vi "initMcode.vi"(5 "PinMode":T1, 6 "CheckMenu":bool, 7 "PinControl":T2=4 items=["4"=4, "10"=10, "13"=13, "14"=14, "15"=15, "53"=53, "54"=54, "55"=55, "56"=56, "57"=57, "58"=58, "66"=66, "67"=67, "68"=68, "69"=69, "77"=77, "78"=78], 8 "error in (no error)":errorcluster, 9 "mCode":T3, 10 "DataVariant":variant, 11 "XuLyDataDisplay in":refnum<class "XuLyDataDisplay.lvclass">) -> (0 "error out":errorcluster, 1 "McodeOut":string, 3 "XuLyDataDisplay out":refnum<class "XuLyDataDisplay.lvclass">)   [LabVIEW 2014, in "LibraryGcode.lvlib" / "XuLyDataDisplay.lvclass"]
uses:
  XuLyDataDisplay.lvclass
  SelectMcode.ctl
  PinControl.ctl
  PinMode.ctl
panel:
  in  "StartingAcceleration":cluster{"P":dbl, "R":dbl, "T":dbl}
  in  "MaxAccel":cluster{"X":dbl, "Y":dbl, "Z":dbl}
  in  "StepPerUnit":cluster{"X":dbl, "Y":dbl, "Z":dbl}
  in  "MaxFeedrate":cluster{"X":dbl, "Y":dbl, "Z":dbl}
  in  "PWM_Out":dbl
  in  "StateBoolean":bool
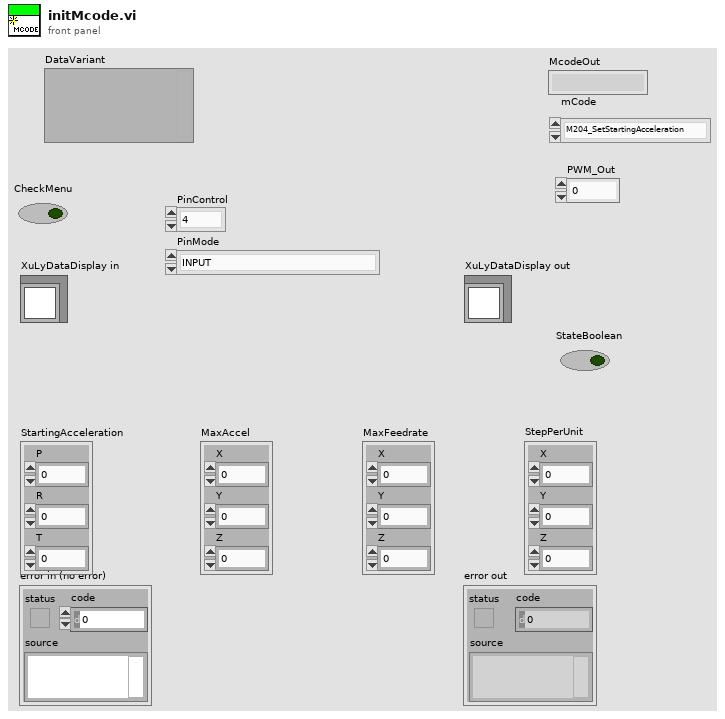
[diagram p1: front panel]
types:
  T1 = typedef "LibraryGcode.lvlib/XuLyDataDisplay.lvclass/PinMode.ctl" = enum16{"INPUT", "OUTPUT", "INPUT_PULLUP", "INPUT_PULLDOWN"}
  T2 = typedef "LibraryGcode.lvlib/XuLyDataDisplay.lvclass/PinControl.ctl" = u16
  T3 = typedef "LibraryGcode.lvlib/XuLyDataDisplay.lvclass/SelectMcode.ctl" = enum16{"M204_SetStartingAcceleration", "M503_ReportSetting", "M500_SaveEprom", "M114_GetPosition", "M92_SetAxisStepPerUnit", "M17_EnableStep", "M18_DisableStep", "M80_PowerOn", "M81_PowerOff", "M112_EMGStop", "M118_SerialPrint", "M226_WaitforPinState", "M400_WaitFinishMove", "M203_SetMaxFeedRate", "M201_SetMaxACCEL", "M380_381_SetSoleNoid_On_Off", "M42_InitPin", "M42_PinControl", "M106_SetFan1", "M106_SetFan2", "M106_SetFan3", "M3_SetSpindle", "M5_OffSpindle", "M999_RestartStop"}
  T4 = typedef "LibraryGcode.lvlib/TypeFirmwareControl.ctl" = enum16{"ScaraMarlin", "CncMarlin", "Mk4Due"}
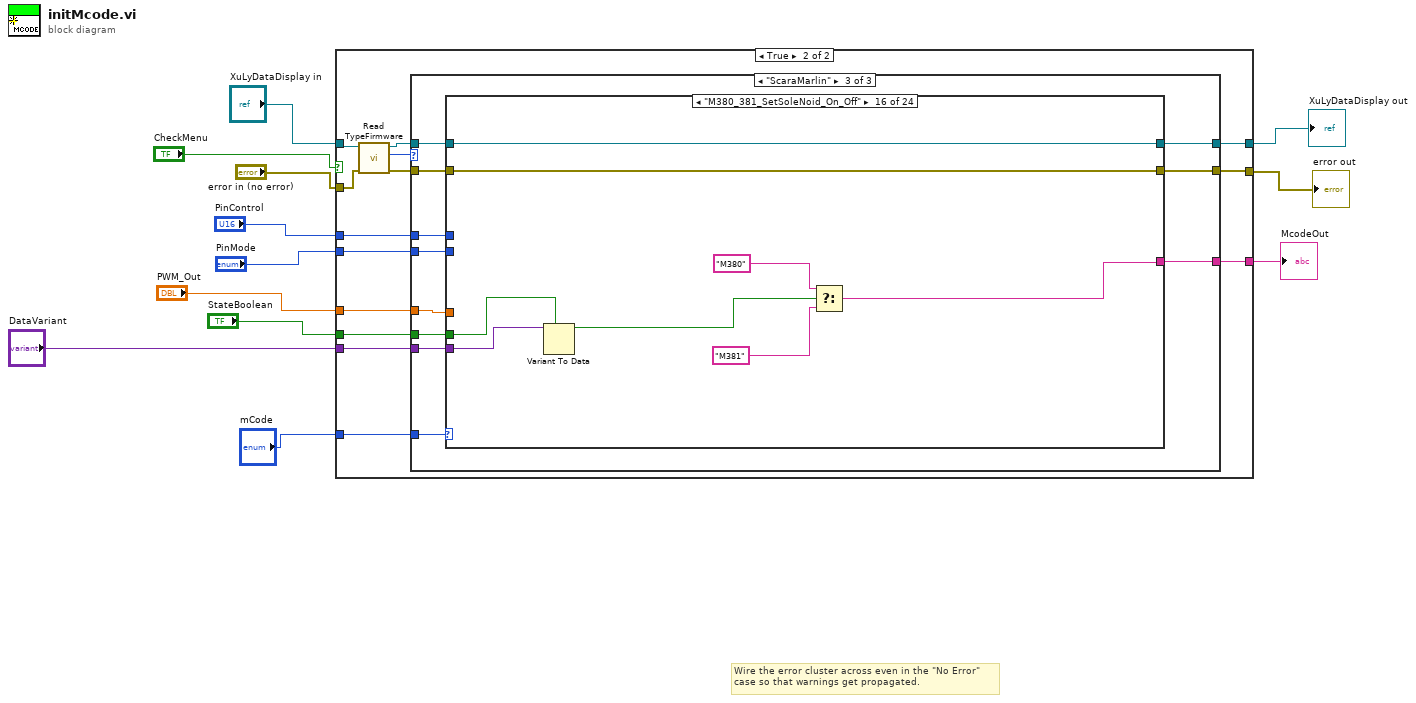
[diagram p0: block diagram]
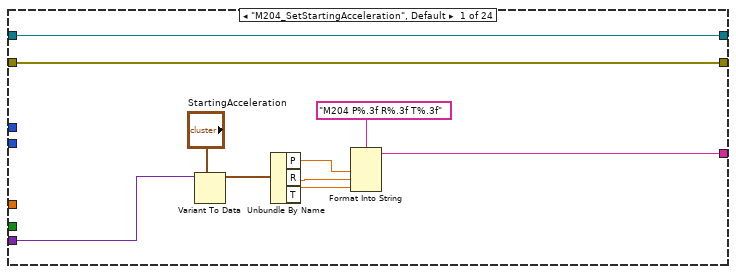
[diagram p5: hidden frame]
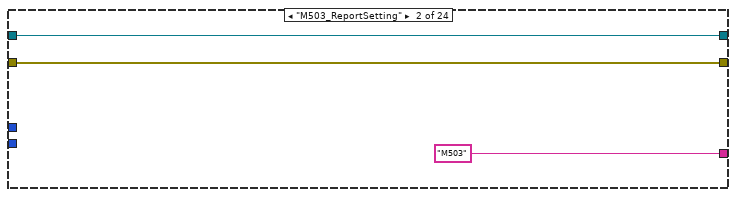
[diagram p6: hidden frame]
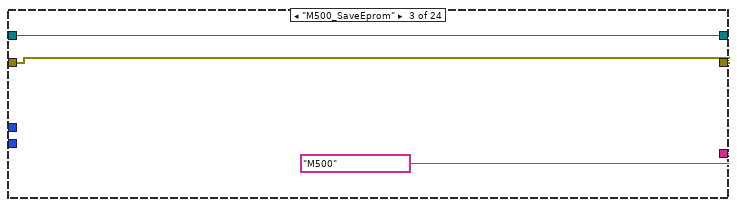
[diagram p7: hidden frame]
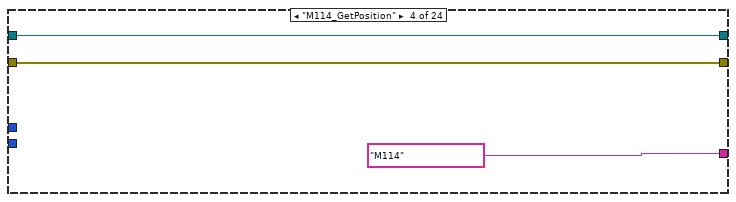
[diagram p8: hidden frame]
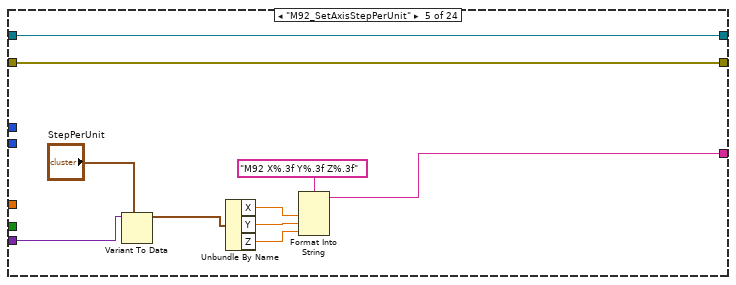
[diagram p9: hidden frame]
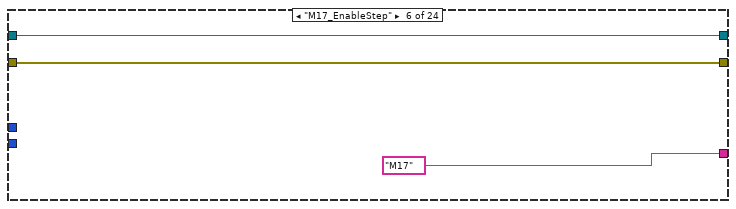
[diagram p10: hidden frame]
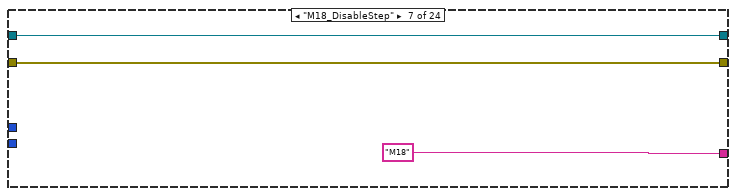
[diagram p11: hidden frame]
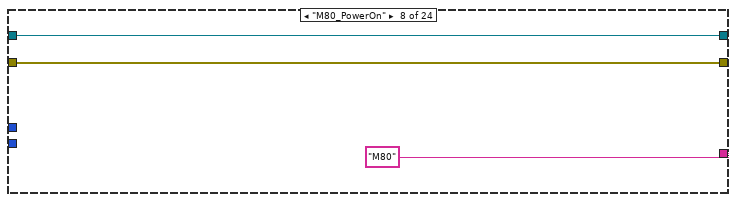
[diagram p12: hidden frame]
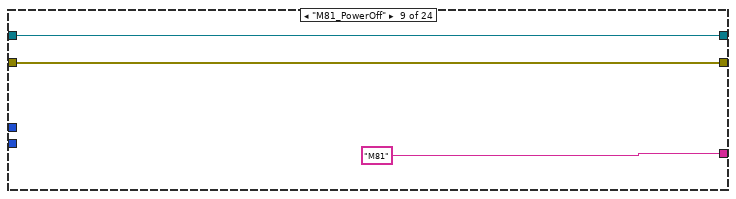
[diagram p13: hidden frame]
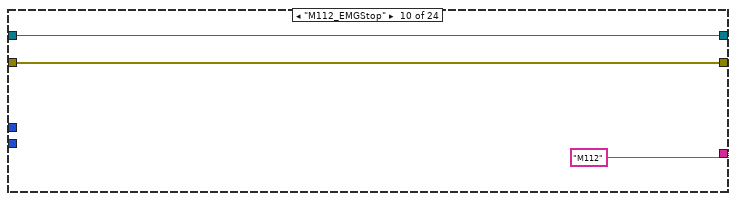
[diagram p14: hidden frame]
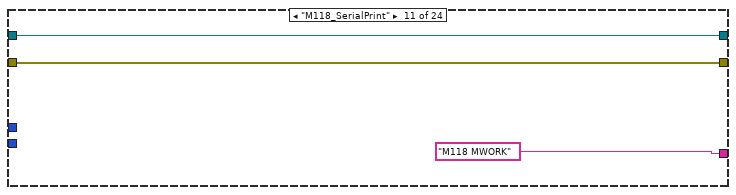
[diagram p15: hidden frame]
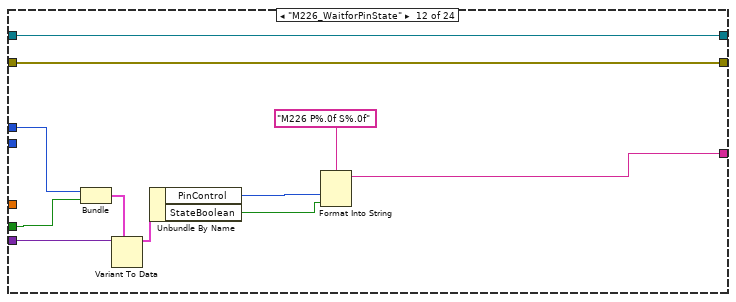
[diagram p16: hidden frame]
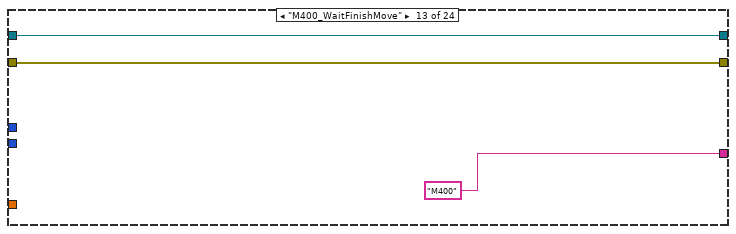
[diagram p17: hidden frame]
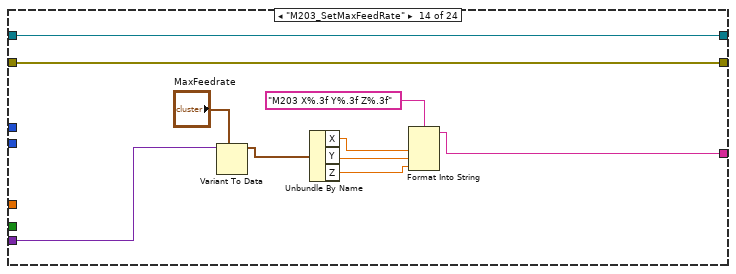
[diagram p18: hidden frame]
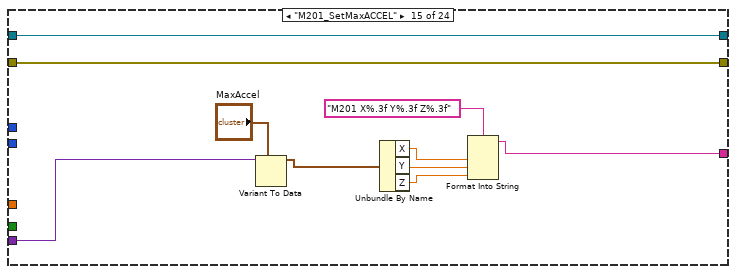
[diagram p19: hidden frame]
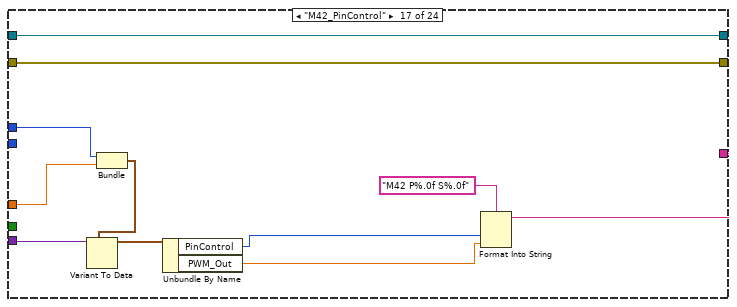
[diagram p20: hidden frame]
diagram:
  # "Wire the error cluster across even in the \"No Error\"\ncase so that warnings get propagated."
  n1 = case shown="True" "CheckMenu" {
    tunnel: [w13 w24] -> w12
    tunnel: [w14 w26] -> w11
    tunnel: "XuLyDataDisplay in" -> [w14 w28]
    tunnel: "mCode" -> [_ w22]
    tunnel: [_ w21] -> w9
    tunnel: "PWM_Out" -> [_ w20]
    tunnel: "PinMode" -> [_ w19]
    tunnel: "PinControl" -> [_ w18]
    tunnel: "DataVariant" -> [_ w17]
    tunnel: "StateBoolean" -> [_ w16]
    tunnel: "error in (no error)" -> [w13 w15]
    frame False {
    }
    frame True {
      n2 = call-dynamic "Read TypeFirmware.vi"("error in (no error)"=w15, "ParameterConf in"=w28) -> ("error out"=w23:errorcluster, "TypeFirmware"=w27:T4, "ParameterConf out"=w25:refnum<class "XuLyDataDisplay.lvclass">)  [unwired: 7 in]
      n3 = case shown="\"ScaraMarlin\"" w27 {
        tunnel: [w30 w32 w40] -> w26
        tunnel: w25 -> [w30 w32 w42]
        tunnel: [w29 w31 w39] -> w24
        tunnel: w23 -> [w29 w31 w41]
        tunnel: w22 -> [_ _ w43]
        tunnel: [_ _ w38] -> w21
        tunnel: w20 -> [_ _ w37]
        tunnel: w19 -> [_ _ w36]
        tunnel: w18 -> [_ _ w35]
        tunnel: w16 -> [_ _ w34]
        tunnel: w17 -> [_ _ w33]
        frame "CncMarlin" {
        }
        frame "Mk4Due" {
        }
        frame "ScaraMarlin" {
          n4 = case shown="\"M380_381_SetSoleNoid_On_Off\"" w43 {
            tunnel: w42 -> [w48 w55 w57 w62 w71 w74 w77 w81 w84 w87 w90 w101 w103 w113 w123 w132 w143 w148 w155 w162 w170 w174 w177 w188]
            tunnel: w41 -> [w47 w56 w58 w61 w70 w73 w76 w80 w83 w86 w89 w99 w102 w112 w122 w131 w142 w147 w154 w161 w169 w173 w176 w187]
            tunnel: [w48 w55 w57 w62 w71 w74 w77 w81 w84 w87 w90 w101 w103 w113 w123 w132 w143 w148 w155 w162 w170 w174 w177 w188] -> w40
            tunnel: [w47 w56 w58 w61 w70 w73 w76 w80 w83 w86 w89 w99 w102 w112 w122 w131 w142 w147 w154 w161 w169 w173 w176 w187] -> w39
            tunnel: [w49 "M503" "M500" "M114" w69 "M17" "M18" "M80" "M81" "M112" "M118 MWORK" w98 "M400" w111 w118 w125 w140 w149 w156 w163 w165 "M5" "M999" w185] -> w38
            tunnel: w37 -> [_ _ _ _ _ _ _ _ _ _ _ _ _ _ _ _ w137 w146 w152 w160 w168 _ _ _]
            tunnel: w36 -> [_ _ _ _ _ _ _ _ _ _ _ _ _ _ _ _ _ _ _ _ _ _ _ w183]
            tunnel: w35 -> [_ _ _ _ _ _ _ _ _ _ _ w96 _ _ _ _ w138 _ _ _ _ _ _ w184]
            tunnel: w34 -> [_ _ _ _ _ _ _ _ _ _ _ w95 _ _ _ w128 _ _ _ _ _ _ _ _]
            tunnel: w33 -> [w44 _ _ _ w64 _ _ _ _ _ _ w97 _ w105 w115 w127 w139 w145 w153 w159 w167 _ _ w181]
            frame "M204_SetStartingAcceleration", Default {
              n5 = Variant To Data(type="StartingAcceleration", Variant=w44) -> (data=w45:cluster{"P":dbl, "R":dbl, "T":dbl})  [unwired: 1 in, 1 out]
              n6 = Unbundle By Name(w45) -> ("P"=w52:dbl, "R"=w51:dbl, "T"=w50:dbl)
              n7 = Format Into String(format string="M204 P%.3f R%.3f T%.3f", w52, w51, w50) -> (resulting string=w49:string)  [unwired: 2 in, 1 out]
            }
            frame "M503_ReportSetting" {
            }
            frame "M500_SaveEprom" {
            }
            frame "M114_GetPosition" {
            }
            frame "M92_SetAxisStepPerUnit" {
              n8 = Variant To Data(type="StepPerUnit", Variant=w64) -> (data=w65:cluster{"X":dbl, "Y":dbl, "Z":dbl})  [unwired: 1 in, 1 out]
              n9 = Unbundle By Name(w65) -> ("X"=w68:dbl, "Y"=w67:dbl, "Z"=w66:dbl)
              n10 = Format Into String(format string="M92 X%.3f Y%.3f Z%.3f", w68, w67, w66) -> (resulting string=w69:string)  [unwired: 2 in, 1 out]
            }
            frame "M17_EnableStep" {
            }
            frame "M18_DisableStep" {
            }
            frame "M80_PowerOn" {
            }
            frame "M81_PowerOff" {
            }
            frame "M112_EMGStop" {
            }
            frame "M118_SerialPrint" {
            }
            frame "M226_WaitforPinState" {
              n11 = Bundle("PinControl"=w96, "StateBoolean"=w95) -> (w94:cluster{"PinControl":T2, "StateBoolean":bool})  [unwired: 1 in]
              n12 = Variant To Data(type=w94, Variant=w97) -> (data=w93:cluster{"PinControl":T2, "StateBoolean":bool})  [unwired: 1 in, 1 out]
              n13 = Unbundle By Name(w93) -> ("PinControl"=w92:T2, "StateBoolean"=w91:bool)
              n14 = Format Into String(format string="M226 P%.0f S%.0f", w92, w91) -> (resulting string=w98:string)  [unwired: 2 in, 1 out]
            }
            frame "M400_WaitFinishMove" {
            }
            frame "M203_SetMaxFeedRate" {
              n15 = Variant To Data(type="MaxFeedrate", Variant=w105) -> (data=w106:cluster{"X":dbl, "Y":dbl, "Z":dbl})  [unwired: 1 in, 1 out]
              n16 = Unbundle By Name(w106) -> ("X"=w110:dbl, "Y"=w109:dbl, "Z"=w108:dbl)
              n17 = Format Into String(format string="M203 X%.3f Y%.3f Z%.3f", w110, w109, w108) -> (resulting string=w111:string)  [unwired: 2 in, 1 out]
            }
            frame "M201_SetMaxACCEL" {
              n18 = Variant To Data(type="MaxAccel", Variant=w115) -> (data=w117:cluster{"X":dbl, "Y":dbl, "Z":dbl})  [unwired: 1 in, 1 out]
              n19 = Unbundle By Name(w117) -> ("X"=w121:dbl, "Y"=w120:dbl, "Z"=w119:dbl)
              n20 = Format Into String(format string="M201 X%.3f Y%.3f Z%.3f", w121, w120, w119) -> (resulting string=w118:string)  [unwired: 2 in, 1 out]
            }
            frame "M380_381_SetSoleNoid_On_Off" {
              n21 = Variant To Data(type=w128, Variant=w127) -> (data=w126:bool)  [unwired: 1 in, 1 out]
              n22 = Select(t="M380", s=w126, f="M381") -> (s? t:f=w125:string)
            }
            frame "M42_PinControl" {
              n23 = Bundle("PinControl"=w138, "PWM_Out"=w137) -> (w136:cluster{"PinControl":T2, "PWM_Out":dbl})  [unwired: 1 in]
              n24 = Variant To Data(type=w136, Variant=w139) -> (data=w135:cluster{"PinControl":T2, "PWM_Out":dbl})  [unwired: 1 in, 1 out]
              n25 = Unbundle By Name(w135) -> ("PinControl"=w134:T2, "PWM_Out"=w133:dbl)
              n26 = Format Into String(format string="M42 P%.0f S%.0f", w134, w133) -> (resulting string=w140:string)  [unwired: 2 in, 1 out]
            }
            frame "M106_SetFan1" {
              n27 = Variant To Data(type=w146, Variant=w145) -> (data=w144:dbl)  [unwired: 1 in, 1 out]
              n28 = Format Into String(format string="M106 P0 S%.0f", w144) -> (resulting string=w149:string)  [unwired: 2 in, 1 out]
            }
            frame "M106_SetFan2" {
              n29 = Variant To Data(type=w152, Variant=w153) -> (data=w151:dbl)  [unwired: 1 in, 1 out]
              n30 = Format Into String(format string="M106 P1 S%.0f", w151) -> (resulting string=w156:string)  [unwired: 2 in, 1 out]
            }
            frame "M106_SetFan3" {
              n31 = Variant To Data(type=w160, Variant=w159) -> (data=w158:dbl)  [unwired: 1 in, 1 out]
              n32 = Format Into String(format string="M106 P2 S%.0f", w158) -> (resulting string=w163:string)  [unwired: 2 in, 1 out]
            }
            frame "M3_SetSpindle" {
              n33 = Variant To Data(type=w168, Variant=w167) -> (data=w166:dbl)  [unwired: 1 in, 1 out]
              n34 = Format Into String(format string="M3 S%.0f", w166) -> (resulting string=w165:string)  [unwired: 2 in, 1 out]
            }
            frame "M5_OffSpindle" {
            }
            frame "M999_RestartStop" {
            }
            frame "M42_InitPin" {
              n35 = Bundle("PinControl"=w184, "PinMode"=w183) -> (w182:cluster{"PinControl":T2, "PinMode":T1})  [unwired: 1 in]
              n36 = Variant To Data(type=w182, Variant=w181) -> (data=w180:cluster{"PinControl":T2, "PinMode":T1})  [unwired: 1 in, 1 out]
              n37 = Unbundle By Name(w180) -> ("PinControl"=w179:T2, "PinMode"=w178:T1)
              n38 = Format Into String(format string="M42 P%.0f M%.0f", w179, w178) -> (resulting string=w185:string)  [unwired: 2 in, 1 out]
            }
          }
        }
      }
    }
  }
  "error out" <- w12
  "XuLyDataDisplay out" <- w11
  "McodeOut" <- w9
